vi "ReadMathcadValues.vi"(10 "Name.Sub":string[](array[string]), 11 "After Var Name":string[](array[string])) -> (3 "Variable Clusters out":T1)   [LabVIEW 2015]
uses:
  Variable cluster.ctl
panel:
  out "Array":string[](array[string])
  out "error IO":errorcluster
  in  "error in":errorcluster
  out "Numeric":i32
  in  "Variable Clusters":T1
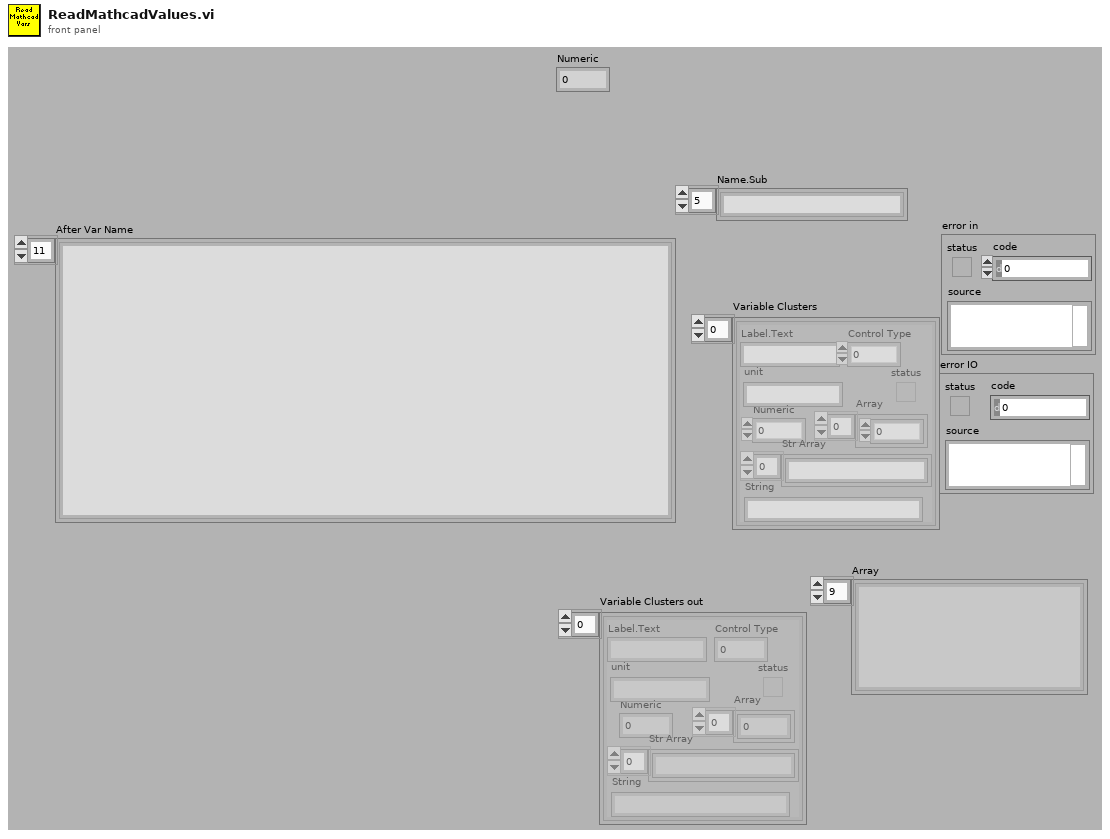
[diagram p1: front panel]
types:
  T1 = typedef "Variable cluster.ctl" = cluster{"Label.Text":string, "Control Type":u32, "Numeric":dbl, "Array":dbl[], "status":bool, "Str Array":string[], "String":string, "unit":string}[]
  T2 = cluster{"Label.Text":string, "Control Type":u32, "Numeric":dbl, "Array":dbl[], "status":bool, "Str Array":string[], "String":string, "unit":string}
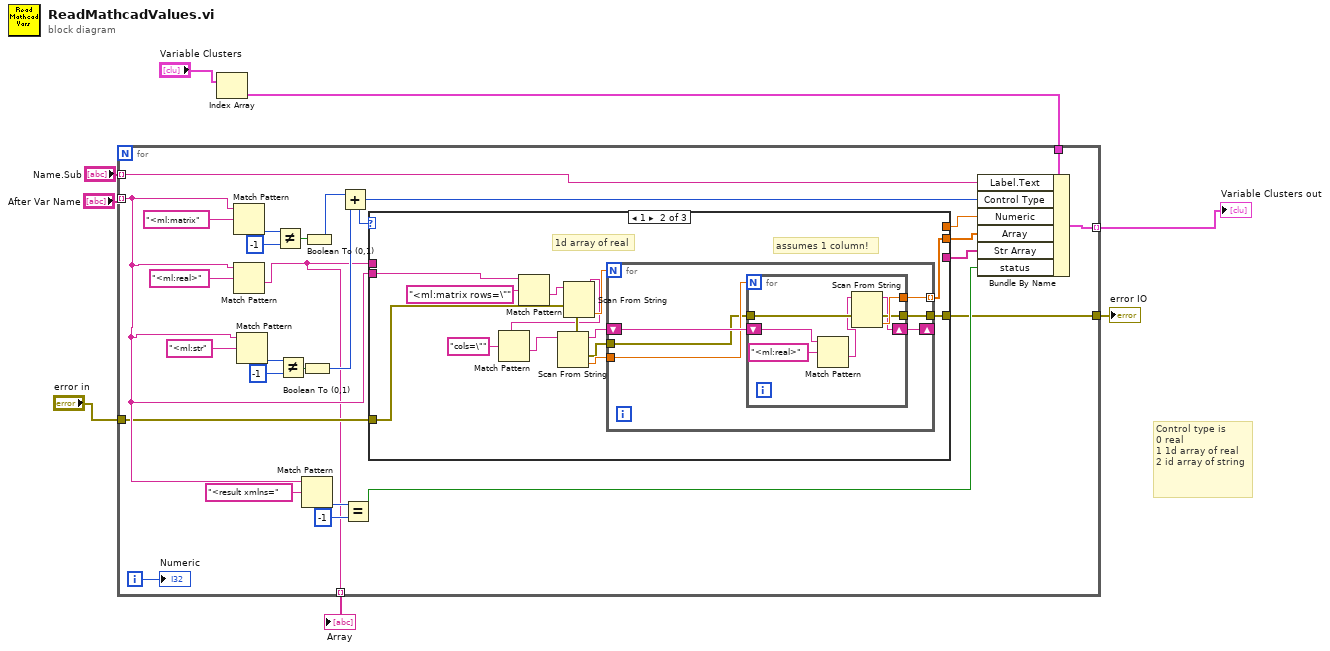
[diagram p0: block diagram]
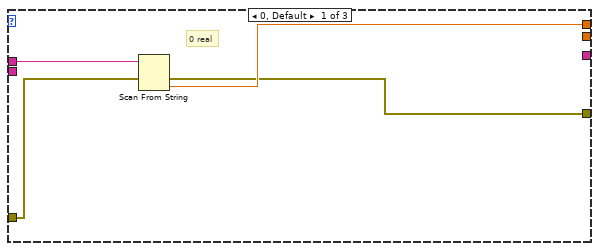
[diagram p2: hidden frame]
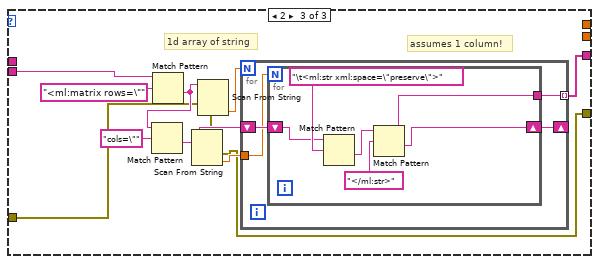
[diagram p3: hidden frame]
diagram:
  # "Control type is\n0 real\n1 1d array of real\n2 id array of string"
  n1 = Index Array(array="Variable Clusters") -> (element=w5:T2)  [unwired: 1 in]
  n2 = for {
    tunnel: "After Var Name" -> [w16] mode=indexing
    tunnel: "Name.Sub" -> [w33] mode=indexing
    tunnel: w5 -> [w35]
    tunnel: [w34] -> w4 mode=indexing
    tunnel: "error in" -> [w11]
    tunnel: [w10] -> w2
    tunnel: [w9] -> w1 mode=indexing
    i -> [w12]
    n3 = Match Pattern(string=w16, regular expression="<ml:matrix") -> (offset past match=w27:i32)  [unwired: 1 in, 3 out]
    n4 = Match Pattern(string=w16, regular expression="<ml:real>") -> (after substring=w9:string)  [unwired: 1 in, 3 out]
    n5 = Match Pattern(string=w16, regular expression="<ml:str") -> (offset past match=w23:i32)  [unwired: 1 in, 3 out]
    n6 = Not Equal?(x=w27, y=-1) -> (x != y?=w21:bool)
    n7 = Not Equal?(x=w23, y=-1) -> (x != y?=w19:bool)
    n8 = Boolean To (0,1)(Boolean=w19) -> (0, 1=w18:i16)
    n9 = Match Pattern(string=w16, regular expression="<result xmlns=") -> (offset past match=w31:i32)  [unwired: 1 in, 3 out]
    n10 = Boolean To (0,1)(Boolean=w21) -> (0, 1=w20:i16)
    n11 = Add(x=w20, y=w18) -> (x+y=w17:i16)
    n12 = Equal?(x=w31, y=-1) -> (x = y?=w29:bool)
    n13 = case shown="1" w17 {
      tunnel: w16 -> [_ w53 w75]
      tunnel: w9 -> [w39 _ _]
      tunnel: [w38 _ _] -> w15
      tunnel: [_ w50 _] -> w14
      tunnel: [_ _ w74] -> w13
      tunnel: w11 -> [w37 w47 w69]
      tunnel: [w36 w44 w67] -> w10
      frame 0, Default {
        # "0 real"
        n14 = Scan From String(input string=w39, error in=w37) -> (error out=w36:errorcluster, output 1=w38:dbl)  [unwired: 3 in, 2 out]
      }
      frame 1 {
        # "assumes 1 column!"
        # "1d array of real"
        n15 = Match Pattern(string=w53, regular expression="<ml:matrix rows=\"") -> (after substring=w43:string)  [unwired: 1 in, 3 out]
        n16 = Scan From String(input string=w43, error in=w47) -> (remaining string=w42:string, error out=w46:errorcluster, output 1=w48:dbl)  [unwired: 3 in, 1 out]
        n17 = Match Pattern(string=w42, regular expression="cols=\"") -> (after substring=w41:string)  [unwired: 1 in, 3 out]
        n18 = Scan From String(input string=w41, error in=w46) -> (remaining string=w40:string, error out=w45:errorcluster, output 1=w49:dbl)  [unwired: 3 in, 1 out]
        n19 = for {
          N: w48 -> [_]
          shift-right: [w59] -> _
          shift-left: w40 -> [w58]
          tunnel: w49 -> [w57]
          tunnel: [w56] -> w50 mode=indexing
          tunnel: w45 -> [w55]
          tunnel: [w54] -> w44
          n20 = for {
            N: w57 -> [_]
            shift-right: [w61] -> w59
            shift-left: w58 -> [w65]
            tunnel: [w64] -> w56
            tunnel: w55 -> [w63]
            tunnel: [w62] -> w54
            n21 = Match Pattern(string=w65, regular expression="<ml:real>") -> (after substring=w60:string)  [unwired: 1 in, 3 out]
            n22 = Scan From String(input string=w60, error in=w63) -> (remaining string=w61:string, error out=w62:errorcluster, output 1=w64:dbl)  [unwired: 3 in, 1 out]
          }
        }
      }
      frame 2 {
        # "assumes 1 column!"
        # "1d array of string"
        n23 = Match Pattern(string=w75, regular expression="<ml:matrix rows=\"") -> (after substring=w71:string)  [unwired: 1 in, 3 out]
        n24 = Match Pattern(string=w71, regular expression="cols=\"") -> (after substring=w70:string)  [unwired: 1 in, 3 out]
        n25 = Scan From String(input string=w71, error in=w69) -> (error out=w68:errorcluster, output 1=w73:dbl)  [unwired: 3 in, 2 out]
        n26 = Scan From String(input string=w70, error in=w68) -> (error out=w67:errorcluster, output 1=w72:dbl)  [unwired: 3 in, 2 out]
        n27 = for {
          N: w73 -> [_]
          shift-right: [w81] -> _
          shift-left: w70 -> [w80]
          tunnel: w72 -> [w79]
          tunnel: [w78] -> w74 mode=indexing
          n28 = for {
            N: w79 -> [_]
            shift-right: [w82] -> w81
            shift-left: w80 -> [w86]
            tunnel: [w85] -> w78
            n29 = Match Pattern(string=w86, regular expression="\t<ml:str xml:space=\"preserve\">") -> (after substring=w84:string)  [unwired: 1 in, 3 out]
            n30 = Match Pattern(string=w84, regular expression="</ml:str>") -> (before substring=w85:string, after substring=w82:string)  [unwired: 1 in, 2 out]
          }
        }
      }
    }
    n31 = Bundle By Name(cluster=w35, "Label.Text"=w33, "Control Type"=w17, "Numeric"=w15, "Array"=w14, "Str Array"=w13, "status"=w29) -> (w34:T2)
    "Numeric" <- w12
  }
  "Variable Clusters out" <- w4
  "error IO" <- w2
  "Array" <- w1
